vi "InitiateMultiPoint.vi"(8 "error in (no error)":errorcluster, 11 "NISTNiPxi6123 in":refnum<class "NiPxi6123.lvclass">) -> (0 "error out":errorcluster, 3 "NISTNiPxi6123 out":refnum<class "NiPxi6123.lvclass">)   [LabVIEW 2014, in "SamplerPlugins.lvlib" / "NiPxi6123.lvclass"]
uses:
  NiPxi6123.lvclass
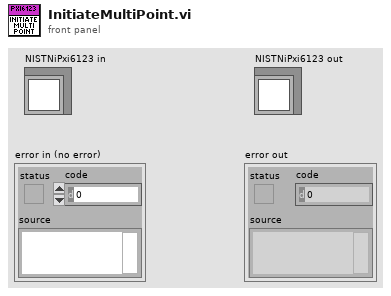
[diagram p1: front panel]
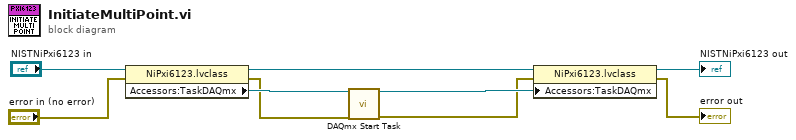
[diagram p0: block diagram]
diagram:
  n1 = property class="NiPxi6123.lvclass"(reference="NISTNiPxi6123 in", error in="error in (no error)") -> (reference out=w7:refnum<class "NiPxi6123.lvclass">, error out=w1:errorcluster, "Accessors:TaskDAQmx"=w2:refnum<k21>)
  n2 = call <vilib>:"DAQmx Start Task.vi"("task/channels in"=w2, "error in"=w1) -> ("task out"=w6:refnum<k21>, "error out"=w5:errorcluster)  [unwired: 12 in]
  n3 = property class="NiPxi6123.lvclass"(reference=w7, error in=w5, "Accessors:TaskDAQmx"=w6) -> (reference out=→"NISTNiPxi6123 out":refnum<class "NiPxi6123.lvclass">, error out=→"error out":errorcluster)
